vi "MB Serial Receive.vi"(7 "Serial Parameters":T1 {"Slave Address" format="%.0x"}, 8 "error in (no error)":errorcluster, 9 "Timeout":u32=10000, 11 "VISA resource name":refnum<visa-resource-name>) -> (0 "error out":errorcluster, 1 "Exception Code":u8 format="%.0x", 2 "Modbus Data Unit":T2={"function"=1, "Data"=[]} {"function" items=["Read Discrete Inputs"=2, "Read Coils"=1, "Write Single Coil"=5, "Write Multiple Coils"=15, "Read Input Register"=4, "Read Holding Registers"=3, "Write Single Register"=6, "Write Multiple Registers"=16, "Read/Write Multiple Registers"=23, "Mask Write Register"=22, "Read FIFO Queue"=24, "Read File Record"=20, "Write File Record"=21, "Read Exception Status"=7, "Diagnostic"=8, "Get Com Event Counter"=11, "Get Com Event Log"=12, "Report Slave ID"=17, "Read Device Identification"=43]; "Data" format="%.0x"}, 3 "VISA resource name out":refnum<visa-resource-name>)   [LabVIEW 2019, in "NI_modbus_upd.lvlib"]
uses:
  NI_modbus_upd.lvlib
  Ctl/MB Modbus Data Unit.ctl
  Modbus Data Unit (PDU)/Function.ctl
panel:
  # "VI Name: MB Serial Receive.vi\nPurpose: Reads a Modbus message."
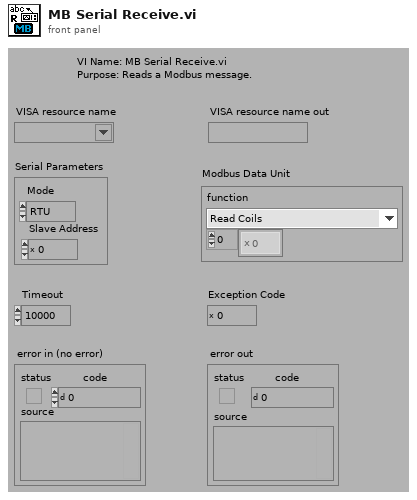
[diagram p1: front panel]
types:
  T1 = cluster{"Mode":enum16{"RTU", "ASCII"}, "Slave Address":u8}
  T2 = typedef "NI_modbus_upd.lvlib/MB Modbus Data Unit.ctl" = cluster{"function":T3, "Data":u8[]}
  T3 = typedef "NI_modbus_upd.lvlib/Function.ctl" = u8
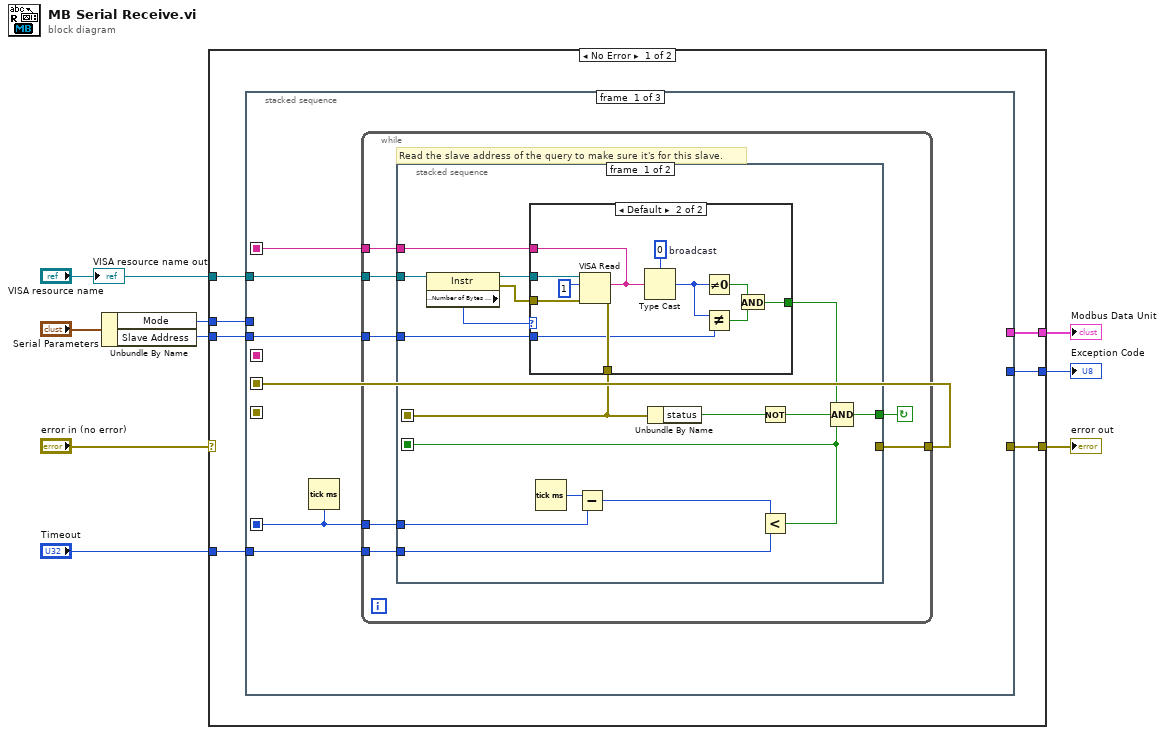
[diagram p0: block diagram]
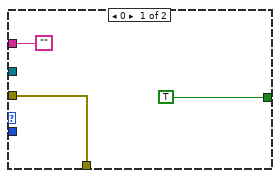
[diagram p2: hidden frame]
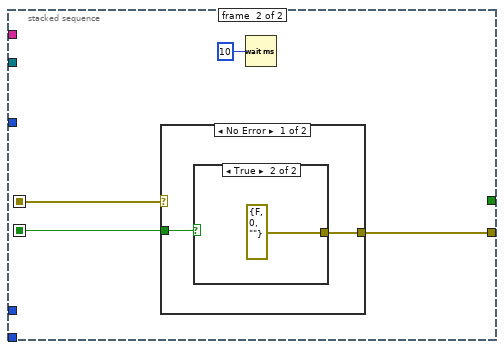
[diagram p3: hidden frame]
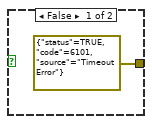
[diagram p4: hidden frame]
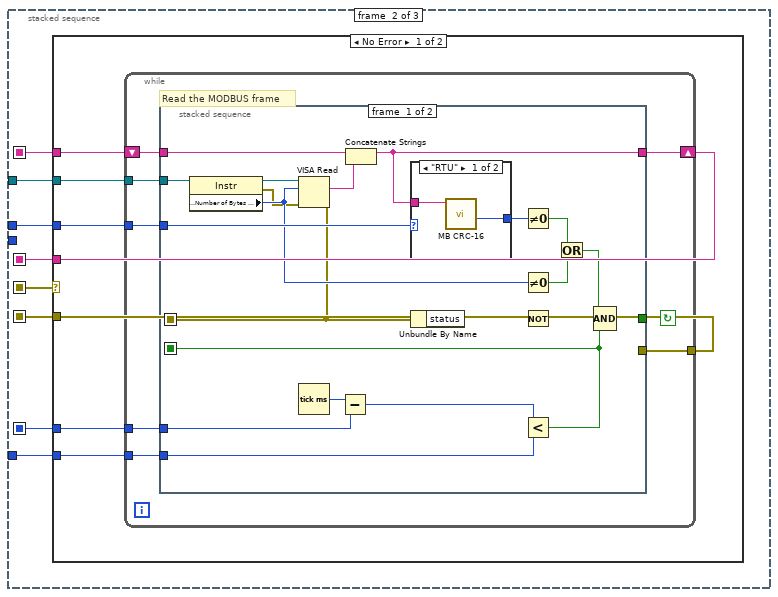
[diagram p6: hidden frame]
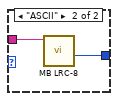
[diagram p7: hidden frame]
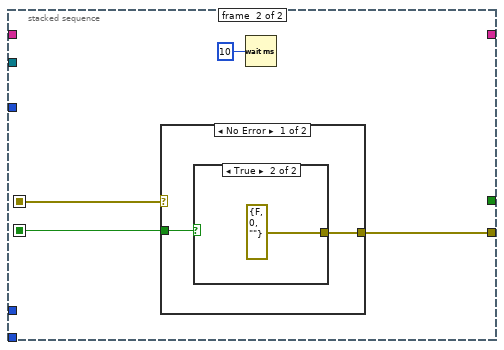
[diagram p8: hidden frame]
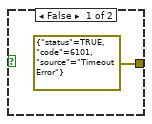
[diagram p9: hidden frame]
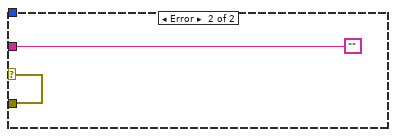
[diagram p11: hidden frame]
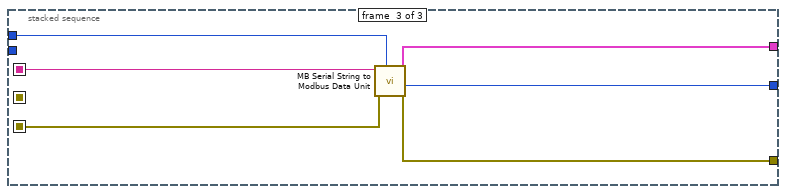
[diagram p12: hidden frame]
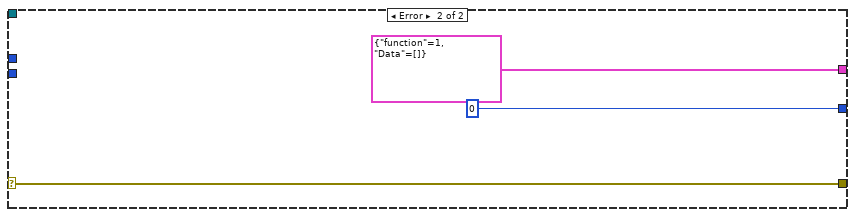
[diagram p13: hidden frame]
diagram:
  n1 = Unbundle By Name("Serial Parameters") -> ("Mode"=w2:enum16{"RTU", "ASCII"}, "Slave Address"=w1:u8)
  n2 = case shown="No Error" "error in (no error)" {
    selector: "error in (no error)" -> [_ w136]
    tunnel: "VISA resource name" -> [w16 _]
    tunnel: w2 -> [w15 _]
    tunnel: [w14 w136] -> w8
    tunnel: [w13 u8 0 ("Exception Code")] -> w6
    tunnel: [w12 T2 {"function"=1, "Data"=[]} ("MODBUS Data Unit")] -> w5
    tunnel: "Timeout" -> [w11 _]
    tunnel: w1 -> [w10 _]
    frame No Error {
      n3 = stacked-sequence {
        seq-local: [_ w74 _] -> [_ _ w131]
        seq-local: [w21 _ _] -> [_ w70 _]
        seq-local: [w19 _ _] -> [_ w72 _]
        seq-local: [_ w71 _] -> [_ _ w128]
        seq-local: [w18 _ _] -> [_ w69 _]
        tunnel: w16 -> [w22 w76 _]
        tunnel: w15 -> [_ w75 w133]
        tunnel: [_ _ w132] -> w14
        tunnel: [_ _ w130] -> w13
        tunnel: [_ _ w129] -> w12
        tunnel: w11 -> [w20 w73 _]
        tunnel: w10 -> [w17 _ _]
        frame #0 {
          n4 = Tick Count (ms)() -> (millisecond timer value=w18:u32)
          n5 = while {
            tunnel: w22 -> [w28]
            tunnel: [w27] -> w21
            tunnel: w20 -> [w26]
            tunnel: [w25] -> w19
            tunnel: w18 -> [w24]
            tunnel: w17 -> [w23]
            stop <- w29 continue-if-true
            # "Read the slave address of the query to make sure it's for this slave."
            n6 = stacked-sequence {
              seq-local: [w38 _] -> [_ w62]
              seq-local: [w37 _] -> [_ w61]
              tunnel: [w45 _] -> w29
              tunnel: w24 -> [w44 _]
              tunnel: w28 -> [w43 _]
              tunnel: [_ w60] -> w27
              tunnel: w26 -> [w36 _]
              tunnel: [w35 _] -> w25
              tunnel: w23 -> [w30 _]
              frame #0 {
                n7 = property class="Instr"(reference=w43) -> (reference out=w42:refnum<visa-resource-name>, error out=w41:errorcluster, "Serial Settings:Number of Bytes at Serial Port"=w34:u32)  [unwired: 1 in]
                n8 = case shown="Default" w34 {
                  tunnel: w42 -> [_ w59]
                  tunnel: w41 -> [w47 w58]
                  tunnel: [w47 w57] -> w38
                  tunnel: ["" w55] -> w35
                  tunnel: [TRUE w50] -> w33
                  tunnel: w30 -> [_ w49]
                  frame 0 {
                  }
                  frame Default {
                    w54 = u8 0  # broadcast
                    n9 = VISA Read(VISA resource name=w59, byte count=u32 1, error in (no error)=w58) -> (read buffer=w55:string, error out=w57:errorcluster)  [unwired: 2 out]
                    n10 = Type Cast(type=w54, x=w55) -> (*(type *) &x=w53:u8)
                    n11 = Not Equal To 0?(x=w53) -> (x != 0?=w52:bool)
                    n12 = Not Equal?(x=w53, y=w49) -> (x != y?=w51:bool)
                    n13 = And(x=w52, y=w51) -> (x .and. y?=w50:bool)
                  }
                }
                n14 = Tick Count (ms)() -> (millisecond timer value=w32:u32)
                n15 = Subtract(x=w32, y=w44) -> (x-y=w31:u32)
                n16 = Unbundle By Name(w38) -> ("status"=w40:bool)
                n17 = Not(x=w40) -> (.not. x?=w39:bool)
                n18 = Less?(x=w31, y=w36) -> (x < y?=w37:bool)
                n19 = Compound Arithmetic op=AND(w33, w39, w37) -> (w45:bool)
              }
              frame #1 {
                n20 = case shown="No Error" w62 {
                  selector: w62 -> [_ w68]
                  tunnel: w61 -> [w65 _]
                  tunnel: [w64 w68] -> w60
                  frame No Error {
                    n21 = case shown="True" w65 {
                      tunnel: [errorcluster {"status"=TRUE, "code"=6101, "source"="Timeout Error"} ("error out") errorcluster {"status"=FALSE, "code"=0, "source"=""} ("error out")] -> w64
                      frame False {
                      }
                      frame True {
                      }
                    }
                  }
                  frame Error {
                  }
                }
                n22 = Wait (ms)(milliseconds to wait=u32 10) -> ()  [unwired: 1 out]
              }
            }
          }
        }
        frame #1 {
          n23 = case shown="No Error" w70 {
            selector: w70 -> [_ w127]
            tunnel: w76 -> [w83 _]
            tunnel: w75 -> [w82 _]
            tunnel: [w81 ""] -> w74
            tunnel: w73 -> [w80 _]
            tunnel: w72 -> [w79 _]
            tunnel: [w78 w127] -> w71
            tunnel: w69 -> [w77 _]
            frame No Error {
              n24 = while {
                tunnel: w82 -> [w90]
                shift-left: w79 -> [w88]
                shift-right: [w85] -> w81
                tunnel: w83 -> [w89]
                tunnel: [w87] -> w78
                tunnel: w80 -> [w86]
                tunnel: w77 -> [w84]
                stop <- w91 continue-if-true
                # "Read the MODBUS frame"
                n25 = stacked-sequence {
                  seq-local: [w95 _] -> [_ w119]
                  seq-local: [w94 _] -> [_ w118]
                  tunnel: [w111 _] -> w91
                  tunnel: w84 -> [w110 _]
                  tunnel: w90 -> [w109 _]
                  tunnel: w89 -> [w104 _]
                  tunnel: w88 -> [w100 _]
                  tunnel: [w98 _] -> w85
                  tunnel: [_ w117] -> w87
                  tunnel: w86 -> [w93 _]
                  frame #0 {
                    n26 = property class="Instr"(reference=w104) -> (reference out=w103:refnum<visa-resource-name>, error out=w101:errorcluster, "Serial Settings:Number of Bytes at Serial Port"=w102:u32)  [unwired: 1 in]
                    n27 = VISA Read(VISA resource name=w103, byte count=w102, error in (no error)=w101) -> (read buffer=w99:string, error out=w95:errorcluster)  [unwired: 2 out]
                    n28 = Tick Count (ms)() -> (millisecond timer value=w112:u32)
                    n29 = Subtract(x=w112, y=w110) -> (x-y=w92:u32)
                    n30 = Concatenate Strings(w100, w99) -> (w98:string)
                    n31 = case shown="\"RTU\"" w109 {
                      tunnel: w98 -> [w114 w116]
                      tunnel: [w113 w115] -> w108
                      frame "RTU" {
                        n32 = call "MB CRC-16.vi"("String"=w114) -> ("CRC-16"=w113:u8)  [unwired: 8 in, 2 out]
                      }
                      frame "ASCII" {
                        n33 = call "MB LRC-8.vi"("String"=w116) -> ("LRC-8"=w115:u8)  [unwired: 8 in, 2 out]
                      }
                    }
                    n34 = Unbundle By Name(w95) -> ("status"=w97:bool)
                    n35 = Not Equal To 0?(x=w108) -> (x != 0?=w107:bool)
                    n36 = Not Equal To 0?(x=w102) -> (x != 0?=w105:bool)
                    n37 = Not(x=w97) -> (.not. x?=w96:bool)
                    n38 = Less?(x=w92, y=w93) -> (x < y?=w94:bool)
                    n39 = Or(x=w107, y=w105) -> (x .or. y?=w106:bool)
                    n40 = Compound Arithmetic op=AND(w106, w96, w94) -> (w111:bool)
                  }
                  frame #1 {
                    n41 = case shown="No Error" w119 {
                      selector: w119 -> [_ w125]
                      tunnel: w118 -> [w122 _]
                      tunnel: [w121 w125] -> w117
                      frame No Error {
                        n42 = case shown="True" w122 {
                          tunnel: [errorcluster {"status"=TRUE, "code"=6101, "source"="Timeout Error"} ("error out") errorcluster {"status"=FALSE, "code"=0, "source"=""} ("error out")] -> w121
                          frame False {
                          }
                          frame True {
                          }
                        }
                      }
                      frame Error {
                      }
                    }
                    n43 = Wait (ms)(milliseconds to wait=u32 10) -> ()  [unwired: 1 out]
                  }
                }
              }
            }
            frame Error {
            }
          }
        }
        frame #2 {
          n44 = call "MB Serial String to Modbus Data Unit.vi"("Mode"=w133, "error in (no error)"=w128, "String"=w131) -> ("error out"=w132:errorcluster, "Exception Code"=w130:u8, "Modbus Data Unit"=w129:T2)  [unwired: 5 in, 1 out]
        }
      }
    }
    frame Error {
    }
  }
  "error out" <- w8
  "Exception Code" <- w6
  "Modbus Data Unit" <- w5
  "VISA resource name out" <- "VISA resource name"
